vi "Get client handle.vi"(8 "error in (no error)":errorcluster, 9 "headers":T1[](array[typedef]), 11 "REST Client in":refnum<class "REST Client.lvclass">) -> (0 "error out":errorcluster, 1 "headers out":T1[](array[typedef]), 2 "Client Handle":refnum<class "Abstract HTTP Client.lvclass">, 3 "REST Client out":refnum<class "REST Client.lvclass">)   [LabVIEW 2020, in "REST Client.lvlib" / "REST Client.lvclass"]
uses:
  REST Client.lvclass
  REST Client.lvclass/REST Client.ctl
  <vilib>/VIPM Community/HTTP Client Plugin - Base/Classes/Abstract HTTP Client/Abstract HTTP Client.lvclass
  HTTP Header.ctl
  <vilib>/NI/Advanced HTTP Client/Header--Combo Box.ctl
  <vilib>/NI/Advanced HTTP Client/Session.lvclass
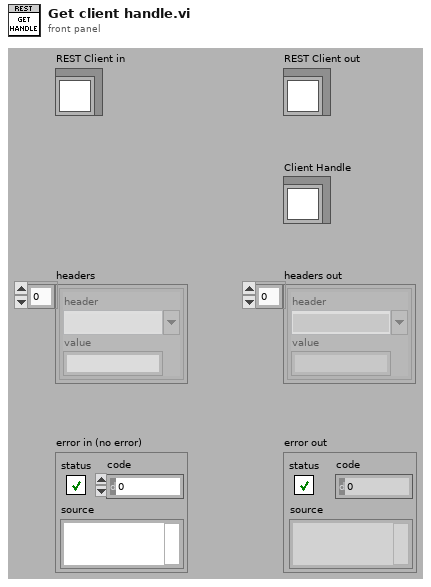
[diagram p1: front panel]
types:
  T1 = typedef "REST Client.lvlib/REST Client.lvclass/HTTP Header.ctl" = cluster{"header":T2, "value":string}
  T2 = typedef "lib_NI_Advanced HTTP Client.lvlib/Session.lvclass/Header--Combo Box.ctl" = string
  T3 = cluster{"HTTP Client Abstract.lvlib:Abstract HTTP Client.lvclass":refnum<class "Abstract HTTP Client.lvclass">, "Default Headers ([JSON])":T1[]}
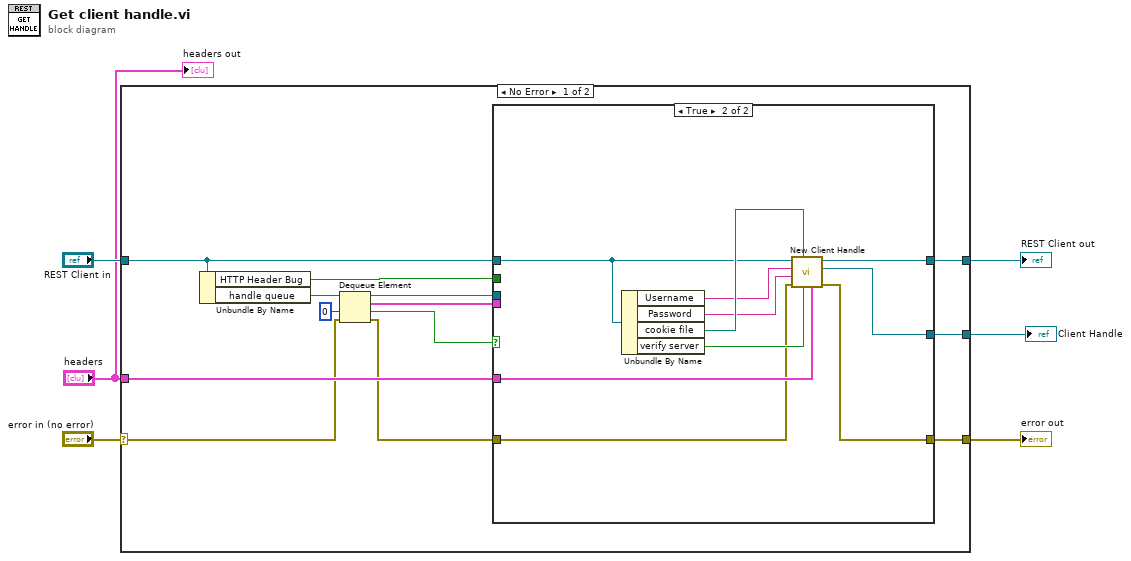
[diagram p0: block diagram]
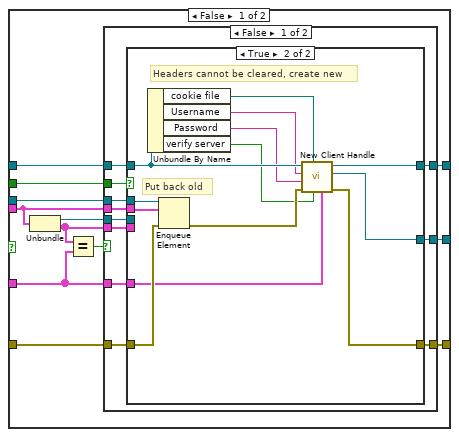
[diagram p2: hidden frame]
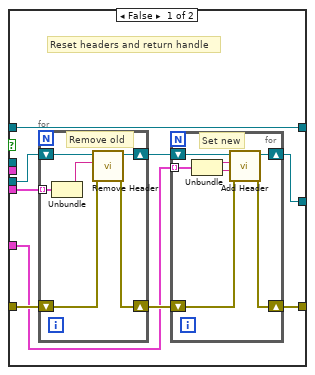
[diagram p3: hidden frame]
diagram:
  n1 = case shown="No Error" "error in (no error)" {
    selector: "error in (no error)" -> [w12 w91]
    tunnel: [w16 w91] -> w5
    tunnel: [w19 w92] -> w3
    tunnel: "REST Client in" -> [w15 w92]
    tunnel: [w17 _] -> w1
    tunnel: "headers" -> [w18 _]
    frame No Error {
      n2 = Unbundle By Name(w15) -> ("HTTP Header Bug"=w8:bool, "handle queue"=w14:refnum<queue>)
      n3 = Dequeue Element(queue=w14, timeout in ms (-1)=0, error in (no error)=w12) -> (queue out=w7:refnum<queue>, element=w9:T3, timed out?=w10:bool, error out=w11:errorcluster)
      n4 = case shown="True" w10 {
        tunnel: [w22 w90] -> w19
        tunnel: w18 -> [w28 w85]
        tunnel: [w27 w84] -> w17
        tunnel: [w26 w83] -> w16
        tunnel: w15 -> [w23 w82]
        tunnel: w11 -> [w25 w81]
        tunnel: w9 -> [w20 _]
        tunnel: w8 -> [w24 _]
        tunnel: w7 -> [w21 _]
        frame False {
          n5 = Unbundle(w20) -> ("HTTP Client Abstract.lvlib:Abstract HTTP Client.lvclass"=w30:refnum<class "Abstract HTTP Client.lvclass">, "Default Headers ([JSON])"=w29:T1[])
          n6 = Equal?(x=w29, y=w28) -> (x = y?=w31:bool)
          n7 = case shown="False" w31 {
            tunnel: w30 -> [w33 w80]
            tunnel: w29 -> [w32 _]
            tunnel: w28 -> [w36 _]
            tunnel: [w34 w80] -> w27
            tunnel: [w35 w79] -> w26
            tunnel: w25 -> [w38 w79]
            tunnel: w24 -> [w42 _]
            tunnel: w23 -> [w41 w78]
            tunnel: [w37 w78] -> w22
            tunnel: w21 -> [w40 _]
            tunnel: w20 -> [w39 _]
            frame False {
              n8 = case shown="True" w42 {
                tunnel: w41 -> [w51 w72]
                tunnel: w40 -> [_ w77]
                tunnel: w39 -> [_ w76]
                tunnel: w38 -> [w48 w75]
                tunnel: [w51 w74] -> w37
                tunnel: w36 -> [w43 w67]
                tunnel: [w45 w66] -> w35
                tunnel: [w46 w65] -> w34
                tunnel: w33 -> [w50 _]
                tunnel: w32 -> [w49 _]
                frame False {
                  # "Reset headers and return handle"
                  n9 = for {
                    shift-right: [w60] -> w44
                    shift-left: w48 -> [w61]
                    shift-right: [w59] -> w47
                    shift-left: w50 -> [w62]
                    tunnel: w49 -> [w64] mode=indexing
                    # "Remove old"
                    n10 = Unbundle(w64) -> ("header"=w63:T2)  [unwired: 1 out]
                    n11 = call-dynamic "Remove Header.vi"("error in (no error)"=w61, "header"=w63, "HTTP Client Abstract in"=w62) -> ("error out"=w60:errorcluster, "HTTP Client Abstract out"=w59:refnum<class "Abstract HTTP Client.lvclass">)  [unwired: 7 in]
                  }
                  n12 = for {
                    shift-right: [w52] -> w45
                    shift-left: w44 -> [w53]
                    shift-right: [w56] -> w46
                    shift-left: w47 -> [w57]
                    tunnel: w43 -> [w58] mode=indexing
                    # "Set new"
                    n13 = Unbundle(w58) -> ("header"=w55:T2, "value"=w54:string)
                    n14 = call-dynamic "Add Header.vi"("error in (no error)"=w53, "value"=w54, "header"=w55, "HTTP Client Abstract in"=w57) -> ("error out"=w52:errorcluster, "HTTP Client Abstract out"=w56:refnum<class "Abstract HTTP Client.lvclass">)  [unwired: 6 in]
                  }
                }
                frame True {
                  # "Put back old"
                  # "Headers cannot be cleared, create new"
                  n15 = Unbundle By Name(w72) -> ("cookie file"=w71:path, "Username"=w70:string, "Password"=w69:string, "verify server"=w68:bool)
                  n16 = Enqueue Element(queue=w77, element=w76, error in (no error)=w75) -> (error out=w73:errorcluster)  [unwired: 1 in, 2 out]
                  n17 = call "New Client Handle.vi"("headers"=w67, "verify server(true)"=w68, "cookie file"=w71, "error in (no error)"=w73, "password"=w69, "username"=w70, "REST Client in"=w72) -> ("error out"=w66:errorcluster, "Client Handle"=w65:refnum<class "Abstract HTTP Client.lvclass">, "REST Client out"=w74:refnum<class "REST Client.lvclass">)  [unwired: 2 in]
                }
              }
            }
            frame True {
              # "Use existing handle"
            }
          }
        }
        frame True {
          n18 = Unbundle By Name(w82) -> ("Username"=w88:string, "Password"=w87:string, "cookie file"=w89:path, "verify server"=w86:bool)
          n19 = call "New Client Handle.vi"("headers"=w85, "verify server(true)"=w86, "cookie file"=w89, "error in (no error)"=w81, "password"=w87, "username"=w88, "REST Client in"=w82) -> ("error out"=w83:errorcluster, "Client Handle"=w84:refnum<class "Abstract HTTP Client.lvclass">, "REST Client out"=w90:refnum<class "REST Client.lvclass">)  [unwired: 2 in]
        }
      }
    }
    frame Error {
    }
  }
  "error out" <- w5
  "REST Client out" <- w3
  "Client Handle" <- w1
  "headers out" <- "headers"
